vi "Output Image Path.vi"(8 "Error In":errorcluster) -> (0 "Error Out":errorcluster, 3 "Image Path":path)   [LabVIEW 2018, in "Image Management.lvlib"]
uses:
  Image Management.lvlib
  Action.ctl
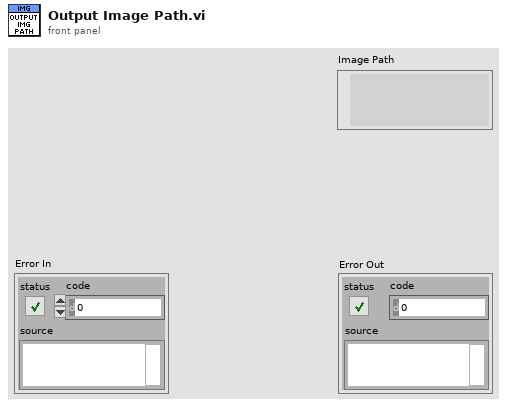
[diagram p1: front panel]
types:
  T1 = typedef "Image Management.lvlib/Action.ctl" = enum16{"Init", "Output Image Path", "Open Image in Default Program", "Find Linespaces", "Get Image Size (pixels)", "Close"}
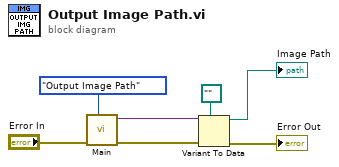
[diagram p0: block diagram]
diagram:
  n1 = call "Main.vi"("Action"=Action."Output Image Path", "Error In"="Error In") -> ("Error Out"=w6:errorcluster, "Output"=w7:variant)  [unwired: 8 in]
  n2 = Variant To Data(error in=w6, type=path "" ("Image Path"), Variant=w7) -> (data=→"Image Path":path, error out=→"Error Out":errorcluster)
